vi "Connection Monitor.vi"(8 "error in (no error)":errorcluster, 11 "RemoteControl.STM in":refnum<class "RemoteControl.STM.lvclass">) -> (0 "error out":errorcluster, 2 "Server out":refnum<class "RemoteControl.lvclass">, 3 "RemoteControl.STM out":refnum<class "RemoteControl.STM.lvclass">)   [LabVIEW 2016, in "RemoteControl.STM.lvclass"]
uses:
  RemoteControl.STM.lvclass
  C:/user/patrick/hg/levylab_inst/lvsrc/SMOs/RemoteControl/RemoteControl.lvclass
  C:/Program Files (x86)/National Instruments/LabVIEW 2016/vi.lib/JKI/JKI SMO/SMO/SMO.lvclass
  RemoteControl/RemoteControl.lvclass
  <vilib>/JKI/JKI SMO/SMO/Typedefs/SMOState --Enum.ctl
  RemoteControl.STM.lvclass/RemoteControl.STM.ctl
  <userlib>/_OpenG.lib/error/error.llb/Filter Error Codes (Array)__ogtk.vi
  <vilib>/JKI/JKI SMO/SMO/SMO.lvclass
panel:
  out "SMO State":T1
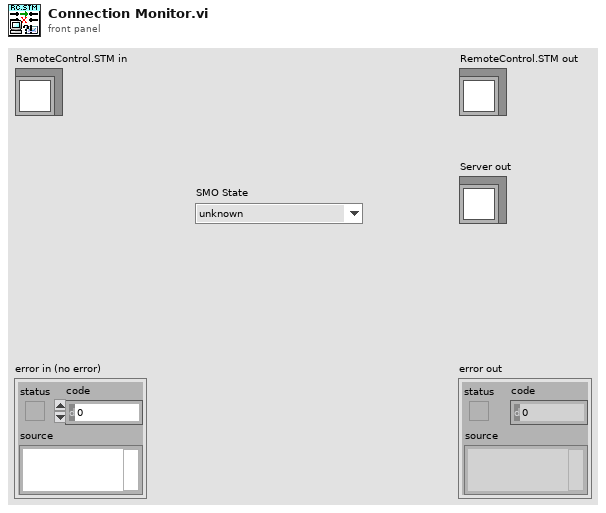
[diagram p1: front panel]
types:
  T1 = typedef "SMO.lvclass/SMOState --Enum.ctl" = enum16{"unknown", "Created", "Started", "Stopped"}
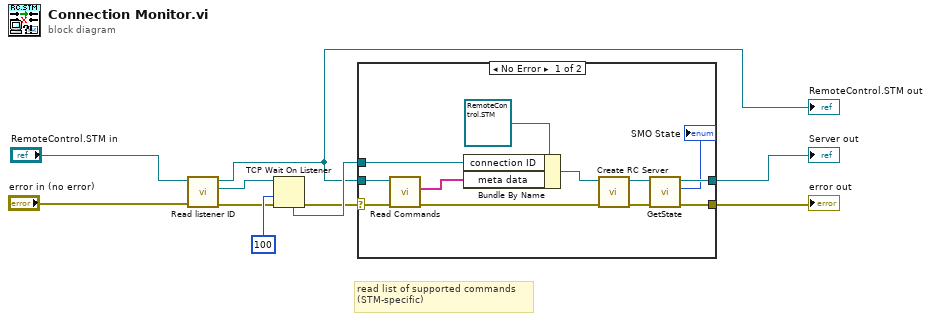
[diagram p0: block diagram]
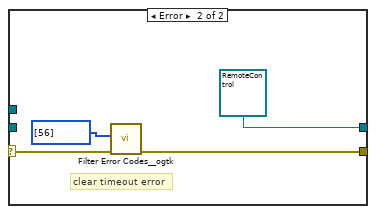
[diagram p2: hidden frame]
diagram:
  # "read list of supported commands\n(STM-specific)"
  n1 = call-dynamic "Read listener ID.vi"("error in (no error)"="error in (no error)", "RemoteControl.STM in"="RemoteControl.STM in") -> ("error out"=w6:errorcluster, "listener ID"=w5:refnum<k5>, "RemoteControl.STM out"=w1:refnum<class "RemoteControl.STM.lvclass">)  [unwired: 7 in]
  "RemoteControl.STM out" <- w1
  n2 = TCP Wait On Listener(8:w6, 9:100 ("timeout ms (wait forever: -1)"), 11:w5) -> (0:w8:errorcluster, 4:w9:refnum<k5>)  [unwired: 1 in, 3 out]
  n3 = case shown="No Error" w8 {
    selector: w8 -> [w18 w25]
    tunnel: w9 -> [w20 _]
    tunnel: [w12 w24] -> w3
    tunnel: [w13 refnum<class "RemoteControl.lvclass"> refnum ("Server out")] -> w4
    tunnel: w1 -> [w19 _]
    frame No Error {
      n4 = call-dynamic "Read Commands.vi"("error in (no error)"=w18, "RemoteControl in"=w19) -> ("error out"=w17:errorcluster, "Commands"=w16:string[])  [unwired: 7 in, 1 out]
      n5 = Bundle By Name(cluster=refnum<class "RemoteControl.STM.lvclass"> refnum ("RemoteControl.STM.lvclass"), "connection ID"=w20, "meta data"=w16) -> (w22:refnum<class "RemoteControl.STM.lvclass">)
      n6 = call-dynamic "Create RC Server.vi"("error in (no error)"=w17, "RemoteControl in"=w22) -> ("error out"=w15:errorcluster, "RemoteControl out"=w14:refnum<class "RemoteControl.STM.lvclass">)  [unwired: 8 in]
      n7 = call <vilib>:"GetState.vi"("error in (no error)"=w15, "SMO"=w14) -> ("error out"=w12:errorcluster, "SMO State"=→"SMO State":T1, "SMO out"=w13:refnum<class "RemoteControl.STM.lvclass">)  [unwired: 7 in]
    }
    frame Error {
      # "clear timeout error"
      n8 = call-poly <userlib>:"Filter Error Codes__ogtk.vi"("Error In"=w25, "Error Codes to Filter"=i32[] [56]) -> ("Error Out"=w24:errorcluster)  [unwired: 7 in, 2 out]
    }
  }
  "error out" <- w3
  "Server out" <- w4
